vi "DSF.Engine.Hardware Info.CPU.Create.vi"(8 "error in (no error)":errorcluster) -> (0 "error out":errorcluster, 3 "CPU Info out":refnum<class "DSF.Engine.Hardware Info.CPU.lvclass">)   [LabVIEW 2017, in "Data Sharing Framework Engine.lvlib" / "DSF.Engine.Hardware Info.CPU.lvclass"]
uses:
  DSF.Engine.Hardware Info.CPU.lvclass
  DSF.Engine.Hardware Info.CPU.lvclass/DSF.Engine.Hardware Info.CPU.ctl
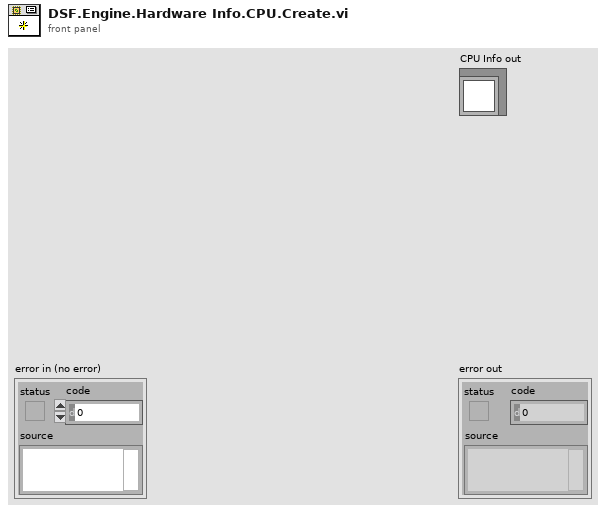
[diagram p1: front panel]
types:
  T1 = cluster{"total cache size":i32, "cache entry size":i32}[]
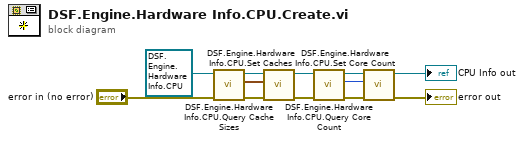
[diagram p0: block diagram]
diagram:
  n1 = call "DSF.Engine.Hardware Info.CPU.Query Cache Sizes.vi"("error in (no error)"="error in (no error)", "CPU Info in"=refnum<class "DSF.Engine.Hardware Info.CPU.lvclass"> refnum) -> ("error out"=w9:errorcluster, "Caches"=w8:T1, "CPU Info out"=w10:refnum<class "DSF.Engine.Hardware Info.CPU.lvclass">)  [unwired: 7 in]
  n2 = call "DSF.Engine.Hardware Info.CPU.Set Caches.vi"("error in (no error)"=w9, "Caches"=w8, "CPU Info in"=w10) -> ("error out"=w6:errorcluster, "CPU Info out"=w7:refnum<class "DSF.Engine.Hardware Info.CPU.lvclass">)  [unwired: 7 in]
  n3 = call "DSF.Engine.Hardware Info.CPU.Query Core Count.vi"("error in (no error)"=w6, "CPU Info in"=w7) -> ("error out"=w4:errorcluster, "Core Count"=w3:i32, "CPU Info out"=w5:refnum<class "DSF.Engine.Hardware Info.CPU.lvclass">)  [unwired: 7 in]
  n4 = call "DSF.Engine.Hardware Info.CPU.Set Core Count.vi"("error in (no error)"=w4, "Core Count"=w3, "CPU Info in"=w5) -> ("error out"=→"error out":errorcluster, "CPU Info out"=→"CPU Info out":refnum<class "DSF.Engine.Hardware Info.CPU.lvclass">)  [unwired: 7 in]
